vi "TestCloneAPI.vi"() -> ()   [LabVIEW 2018, in "DigitizerModule.lvlib"]
uses:
  DigitizerModule.lvlib
  DigitizerPlugins/DigitizerBaseClass/Typedefs/WfrmAttributes.ctl
  TestInfo.ctl
  <userlib>/NIST/ModuleAdminLib/CloneRegistration/CloneRegistration.lvclass
  <userlib>/NIST/ModuleAdminLib/ModuleAdmin/ModuleAdmin.lvclass/ModuleAdmin.ctl
  <userlib>/NIST/ModuleAdminLib/ModuleAdmin/ModuleAdmin.lvclass
  PublicAPI/Arguments/Broadcasts/clDidInit.ctl
  PublicAPI/Arguments/Requests/clStopArgument.ctl
  <userlib>/NIST/ModuleAdminLib/ModuleAdmin/Accessors/Read CloneRegRef.vi
  <userlib>/NIST/ModuleAdminLib/ModuleAdmin/Accessors/Write CloneRegRef.vi
  DigitizerPlugins/DigitizerBaseClass/DigitizerBase.lvclass
panel:
  in  "btnClose":bool
  out "Attributes":T1[][](array[typedef])
  out "Timing":cluster{"Time Stamp":timestamp, "dt":dbl}[][](array[cluster])
  in  "btnAbort":bool
  in  "btnClear":bool
  in  "btnCfgTrig":bool
  in  "btnCfgAquis":bool
  in  "btnCfgChan":bool
  out "Waveform Chart":waveform(dbl)[](graph)
  in  "btnInitialize":bool
  in  "btnReadWfrm":bool
  in  "btnFetch":bool
  in  "btnPref":bool
  in  "Show Panel":bool=TRUE
  in  "Plugin Type":u16(ring) items=["Agilent3458", "IVI Digitizer", "AbsPhase_Voltage", "Analyse Waveforms", "Debug", "INRiM_3Ch", "INRiM_4Ch", "INRiM_5Ch", "INRiM_6Ch", "INRM_1Ch", "Offset Trigger", "PMU Cal", "PRS_FGen", "Simulation"]
  in  "btnLoadPlugin":bool
  out "Path":path
  in  "btnRequestINIPath":bool
  in  "btnRemove":bool
  out "Status Log":string
  out "Active Modules (Array)":string[](array[string])
  in  "btnAdd":bool
  in  "btnStop":bool
  in  "Select Module":i32(ring)=-1 caption="Select Module to send Request" items=["All"=-1]
  # "Hidden"
  # "Visible"
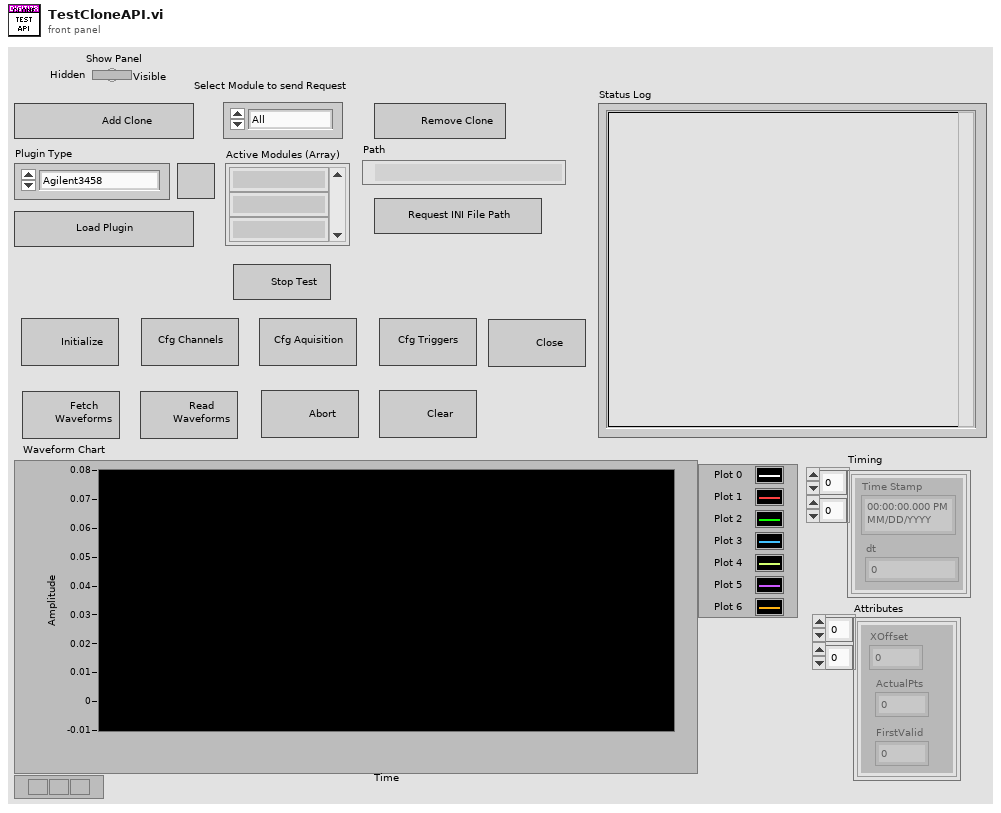
[diagram p1: front panel]
types:
  T1 = typedef "DigitizerPlugins.lvlib/DigitizerBase.lvclass/WfrmAttributes.ctl" = cluster{"XOffset":dbl, "ActualPts":i64, "FirstValid":i64}
  T2 = typedef "DigitizerModule.lvlib/TestInfo.ctl" = cluster{"PluginIniFilePaths":path[]}
  T3 = typedef "DigitizerModule.lvlib/clBroadcastEvents.ctl" = cluster{"DidInit":refnum<user-event>, "StatusUpdate":refnum<user-event>, "ErrorReport":refnum<user-event>, "DidStop":refnum<user-event>, "PathToINI":refnum<user-event>, "Channels":refnum<user-event>, "Acq":refnum<user-event>, "Trigger":refnum<user-event>, "Waveforms":refnum<user-event>}
  T4 = typedef "DigitizerModule.lvlib/clDidInit.ctl" = cluster{"Init?":bool, "ModuleAdmin":refnum<class "ModuleAdmin.lvclass">}
  T5 = typedef "DigitizerModule.lvlib/clStopArgument.ctl" = cluster{"Exit via Stop Module Req?":bool, "Wait for Module to stop?":bool, "ModuleAdmin":refnum<class "ModuleAdmin.lvclass">}
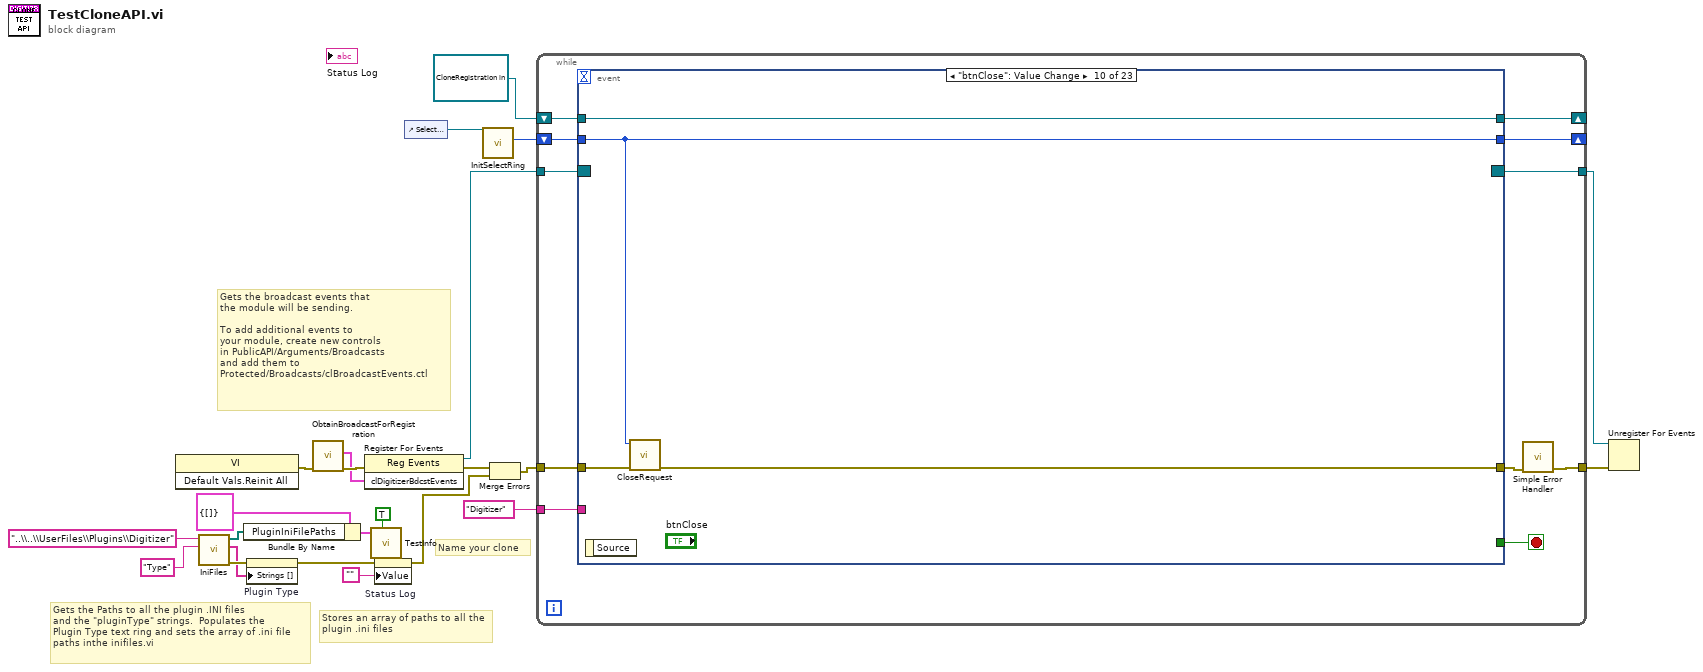
[diagram p0: block diagram]
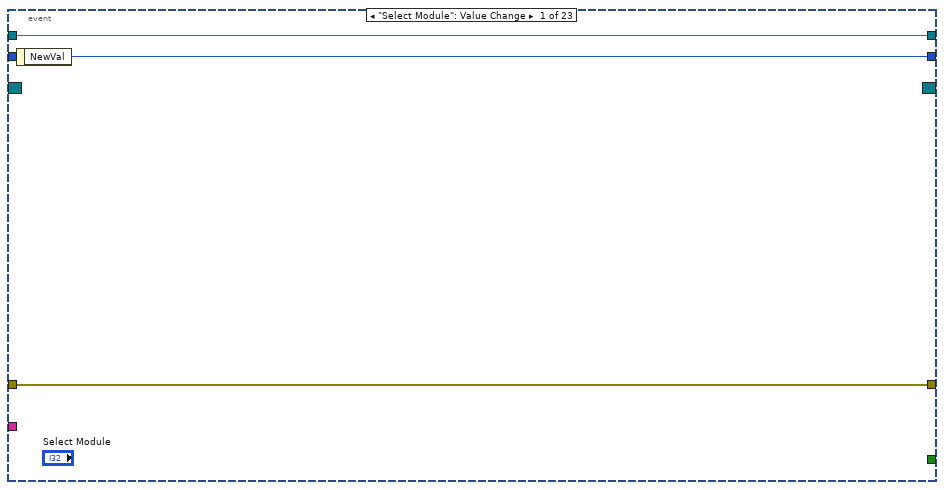
[diagram p2: hidden frame]
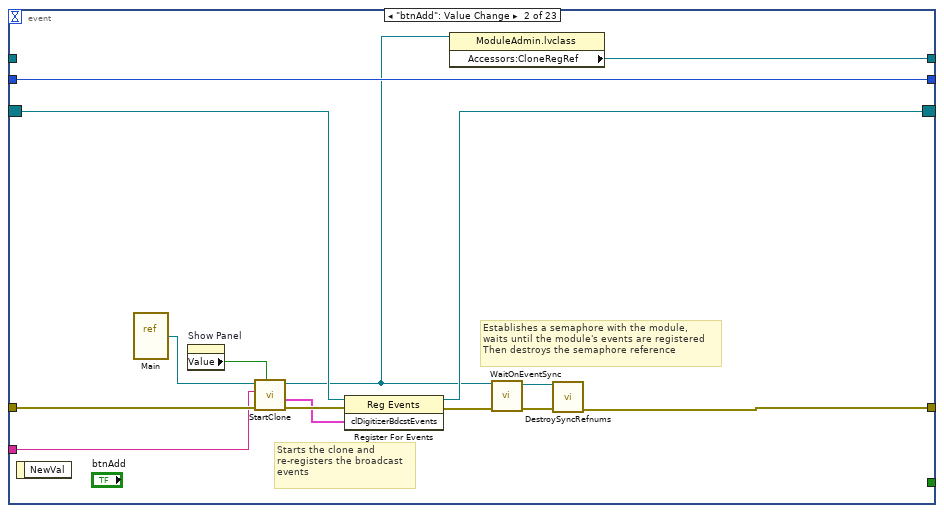
[diagram p3: hidden frame]
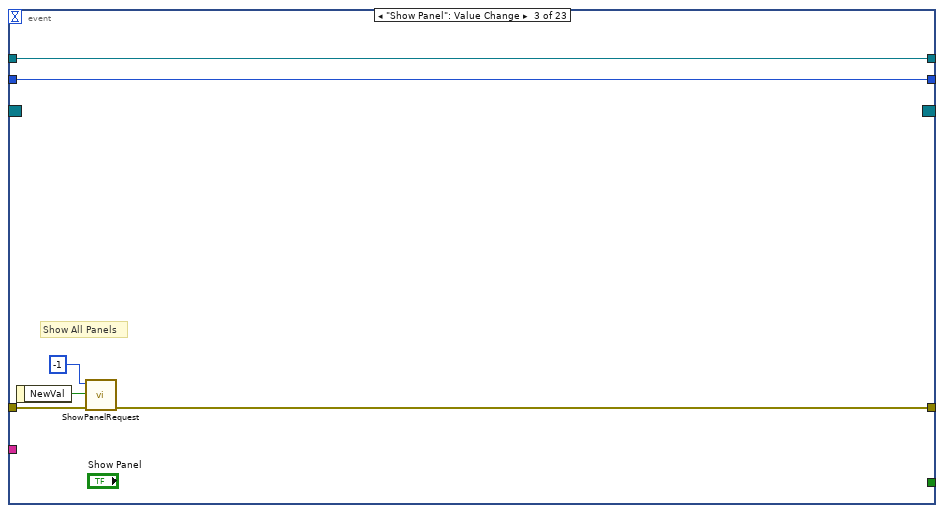
[diagram p4: hidden frame]
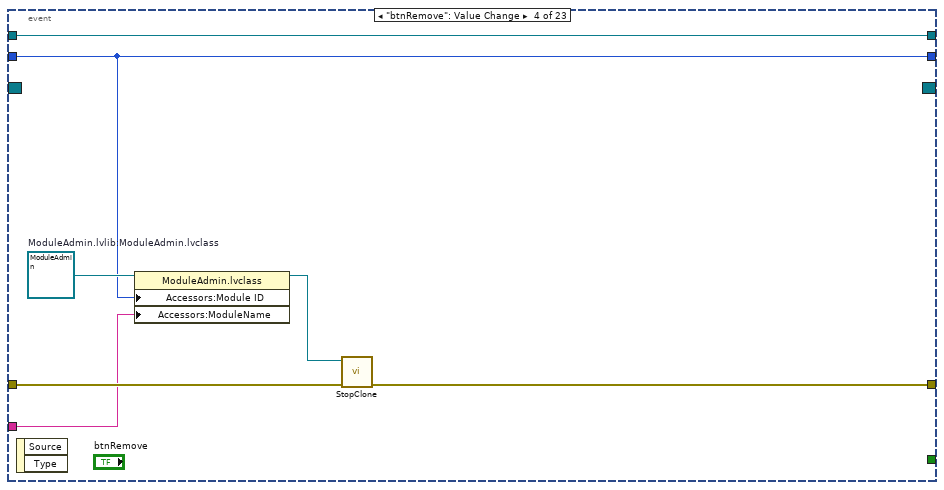
[diagram p5: hidden frame]
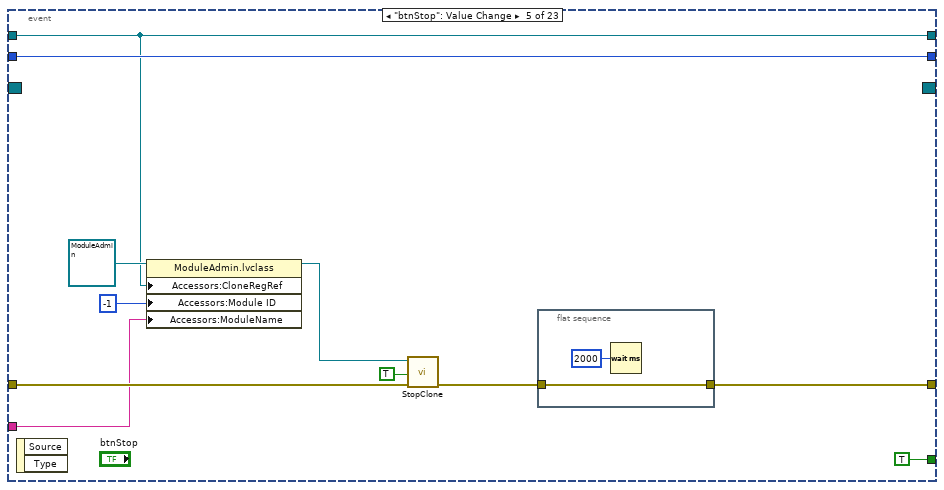
[diagram p6: hidden frame]
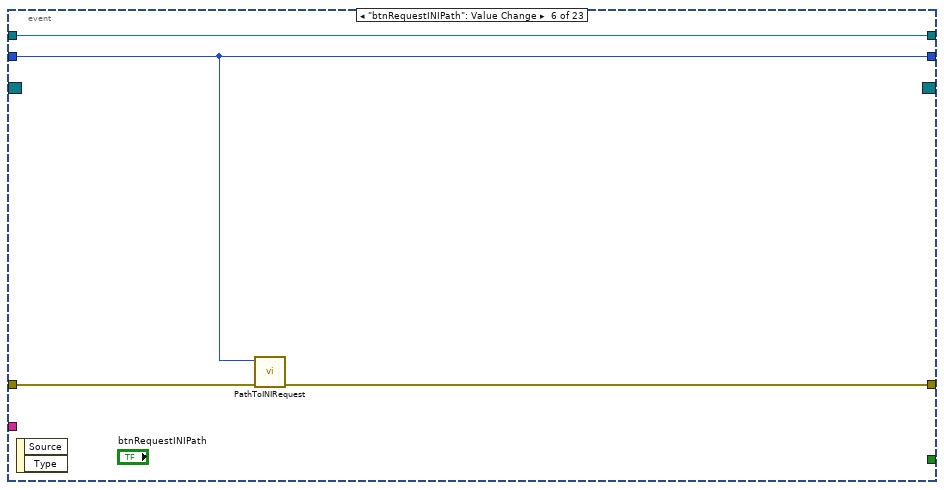
[diagram p7: hidden frame]
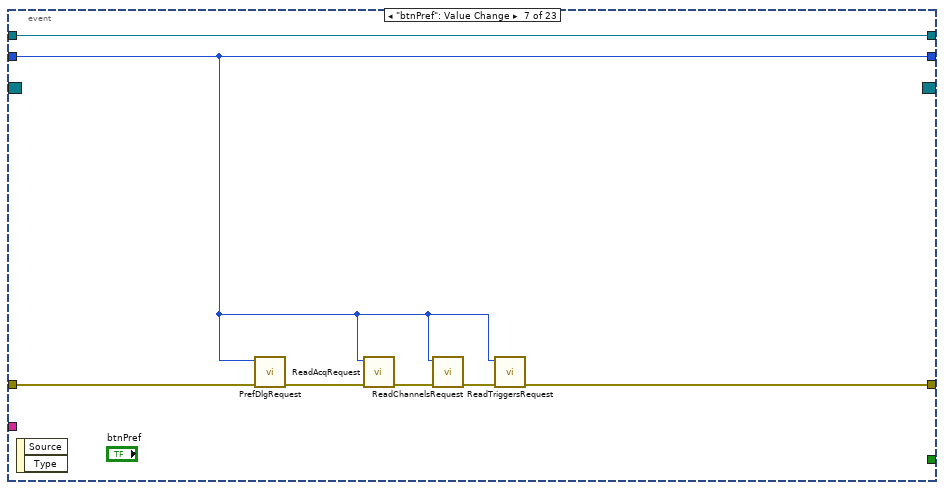
[diagram p8: hidden frame]
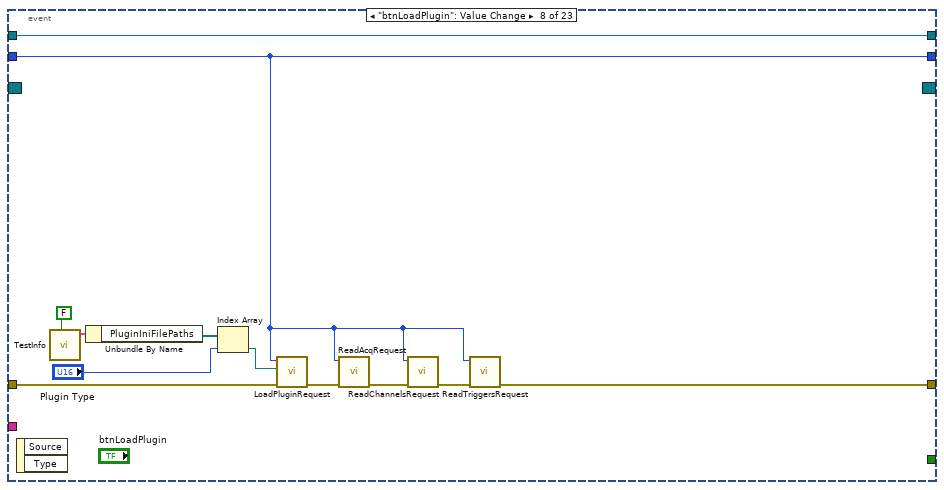
[diagram p9: hidden frame]
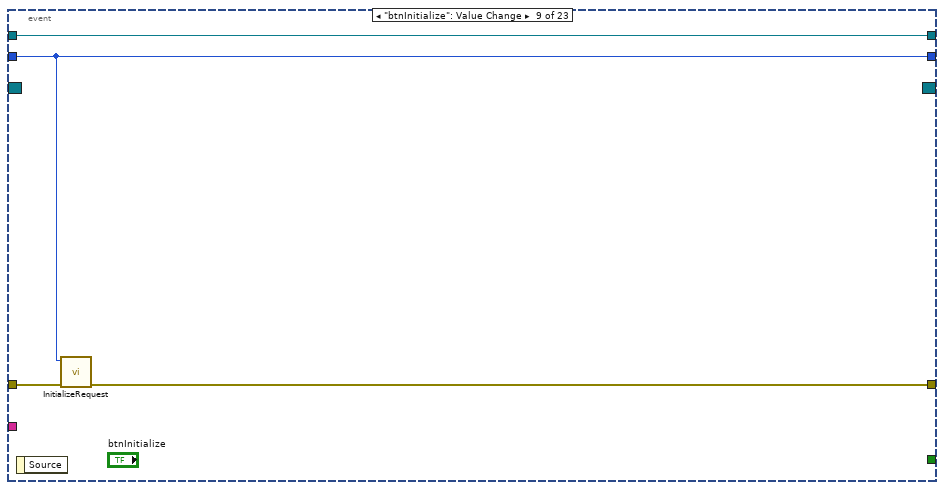
[diagram p10: hidden frame]
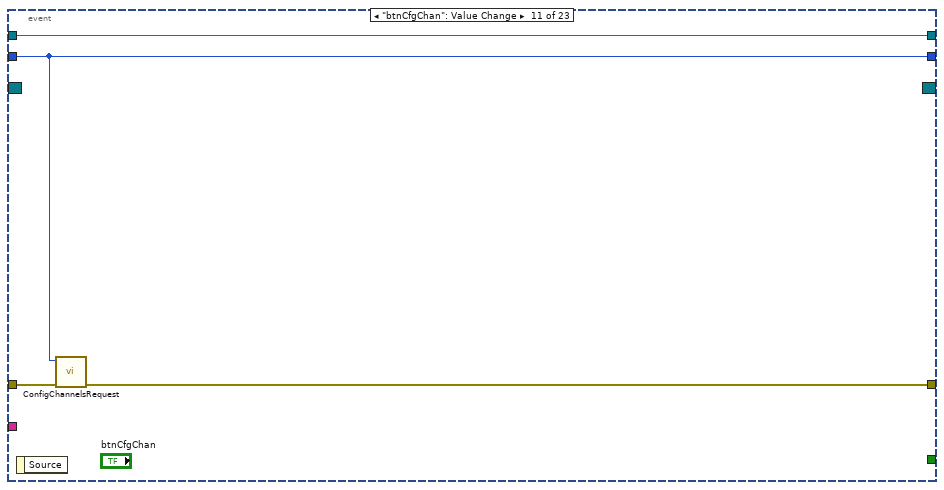
[diagram p11: hidden frame]
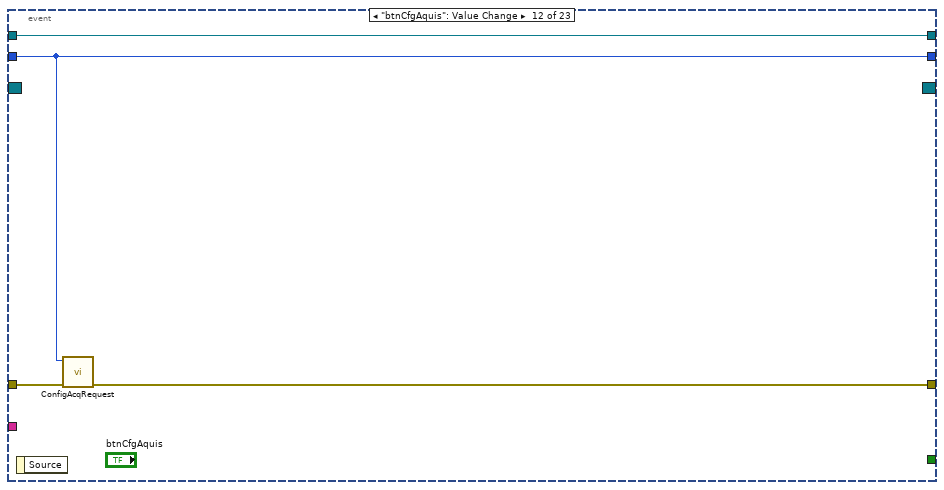
[diagram p12: hidden frame]
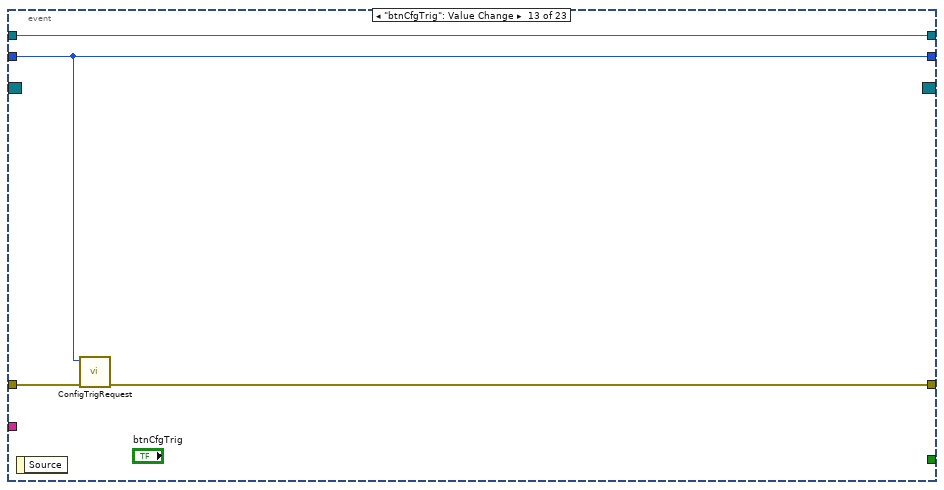
[diagram p13: hidden frame]
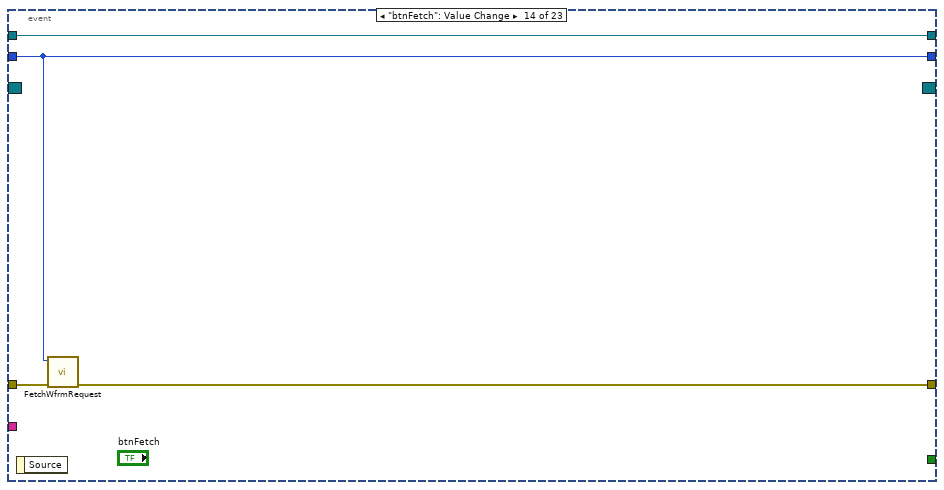
[diagram p14: hidden frame]
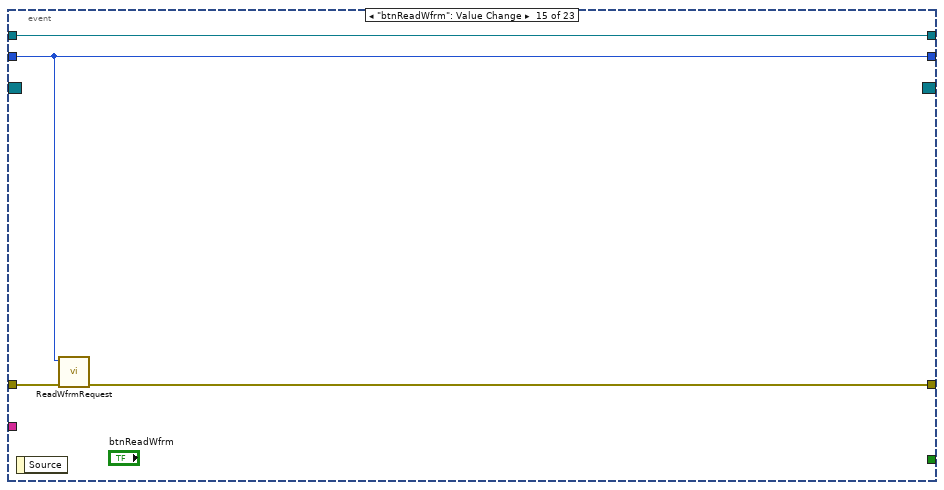
[diagram p15: hidden frame]
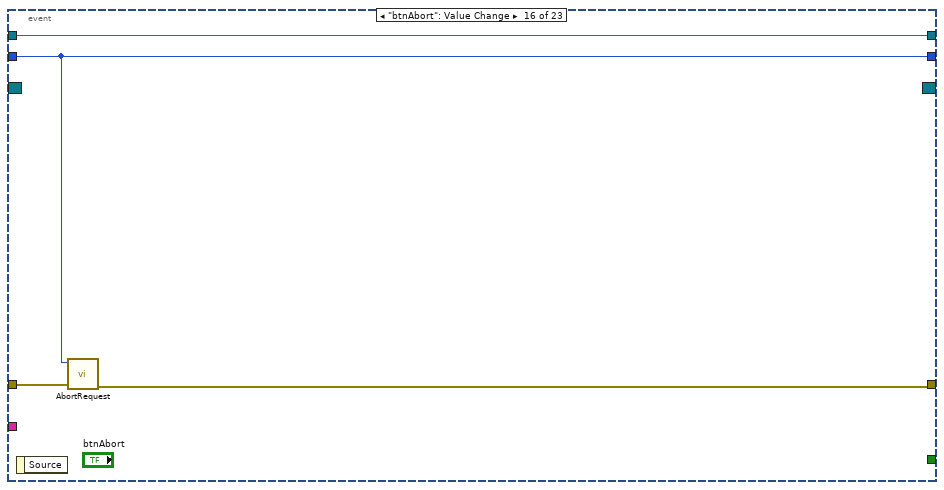
[diagram p16: hidden frame]
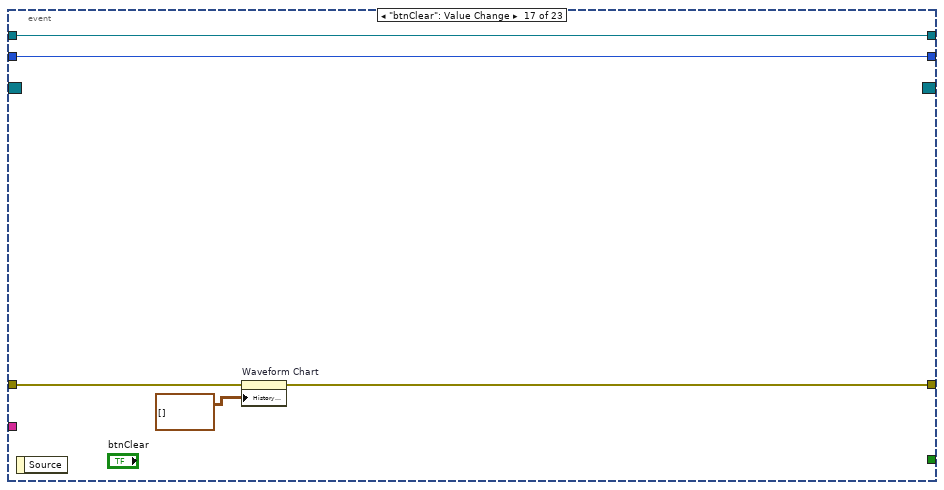
[diagram p17: hidden frame]
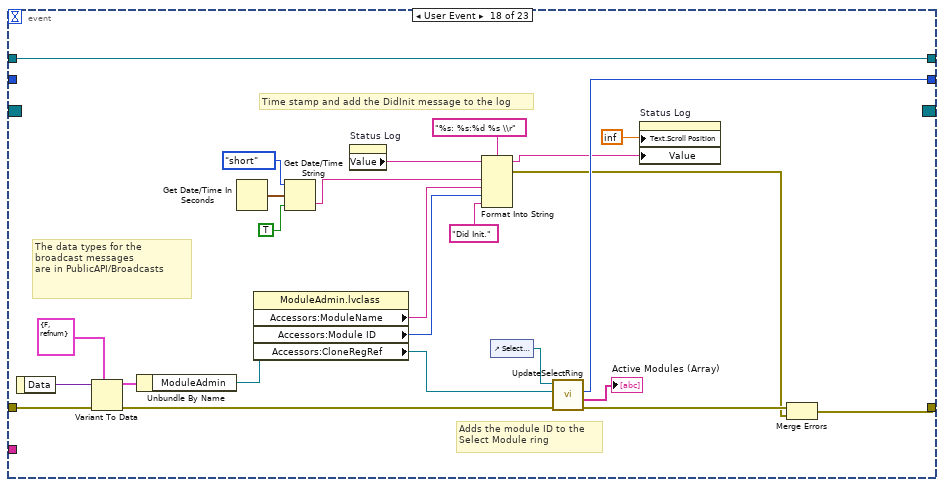
[diagram p18: hidden frame]
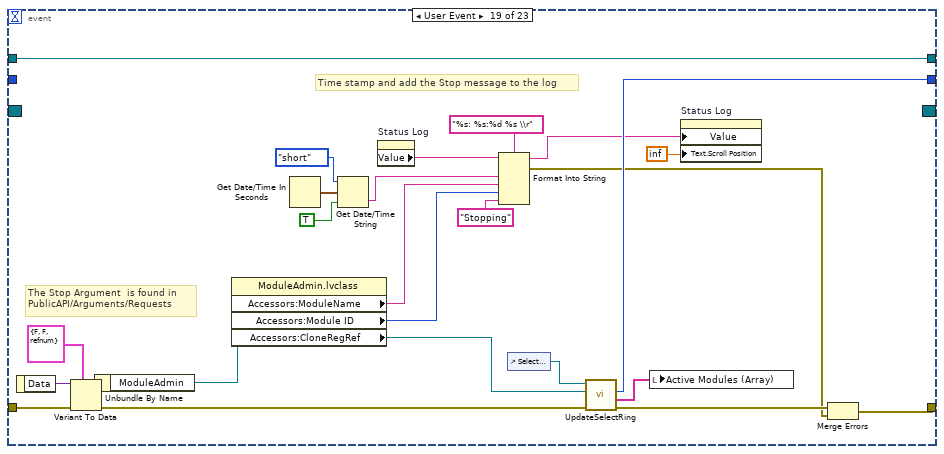
[diagram p19: hidden frame]
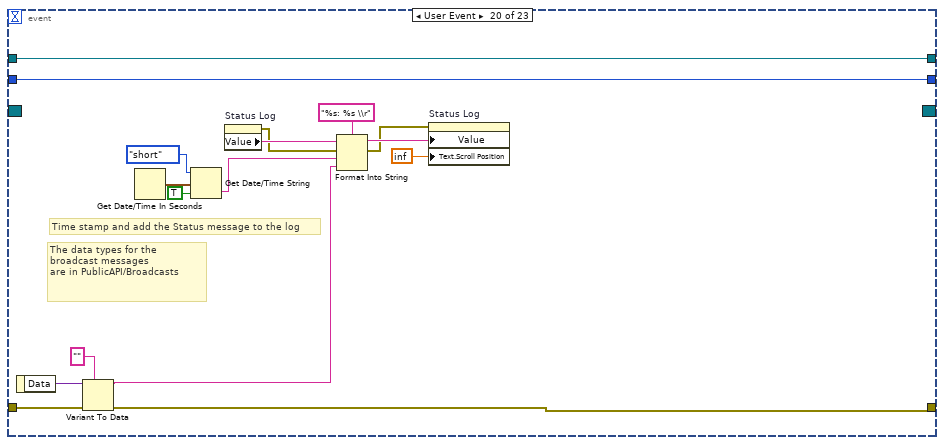
[diagram p20: hidden frame]
diagram:
  # "Stores an array of paths to all the plugin .ini files"
  # "Gets the Paths to all the plugin .INI files\nand the \"pluginType\" strings.  Populates the \nPlugin Type text ring and sets the array of .ini file\npaths inthe inifiles.vi"
  # "Name your clone"
  # "Gets the broadcast events that\nthe module will be sending.\n\nTo add additional events to\nyour module, create new controls\nin PublicAPI/Arguments/Broadcasts\nand add them to\nProtected/Broadcasts/clBroadcastEvents.ctl"
  n1 = invoke class="VI" method="Default Vals.Reinit All"() -> (error out=w21:errorcluster)  [unwired: 3 in, 2 out]
  n2 = call "IniFiles.vi"("iniKey"="Type", "name or relative path"="..\\..\\UserFiles\\Plugins\\Digitizer") -> ("error out"=w15:errorcluster, "Types"=w14:string[], "IniFilePaths"=w13:path[])  [unwired: 7 in]
  n3 = Bundle By Name(cluster=T2 {"PluginIniFilePaths"=[]} ("TestInfo"), "PluginIniFilePaths"=w13) -> (w12:T2)
  n4 = property on="Plugin Type" class="Ring (strict)"(error in=w15, "Strings []"=w14) -> (error out=w3:errorcluster)  [unwired: 1 in, 1 out]
  n5 = call "ObtainBroadcastForRegistration.vi"("error in (no error)"=w21) -> ("error out"=w20:errorcluster, "clDigitizerBdcstEvents"=w19:T3)  [unwired: 9 in]
  n6 = register-events(error in=w20, w19) -> (reference out=w17:refnum<event-registration>, error out=w18:errorcluster)  [unwired: 1 in]
  n7 = call "TestInfo.vi"("Set (f)"=TRUE, "TestInfo 2"=w12) -> ()  [unwired: 9 in, 1 out]
  n8 = property on="Status Log" class="Str"(error in=w3, "Value"="") -> (error out=w2:errorcluster)  [unwired: 1 in, 1 out]
  n9 = control-ref of="Select Module"() -> (w23:refnum<vi>)
  n10 = call "InitSelectRing.vi"("Ring Refnum"=w23) -> ("Module Ring Value"=w22:i32)  [unwired: 9 in, 1 out]
  n11 = Merge Errors(w18, w2) -> (w10:errorcluster)
  n12 = while {
    shift-right: [w33] -> _
    shift-left: w22 -> [w34]
    tunnel: w10 -> [w31]
    tunnel: w17 -> [w28]
    tunnel: [w29] -> w6
    tunnel: "Digitizer" ("ModuleName") -> [w27]
    tunnel: [w26] -> w5
    shift-right: [w25] -> _
    shift-left: refnum<data-value> refnum ("Accessors:CloneRegRef") -> [w24]
    stop <- w32 stop-if-true
    n13 = event shown="[9] \"btnClose\": Value Change" {
      selector: w28 -> [_ w44 _ _ _ _ _ _ _ _ _ _ _ _ _ _ _ _ _ _ _ _ _]
      dyn-events: [_ w43 _ _ _ _ _ _ _ _ _ _ _ _ _ _ _ _ _ _ _ _ _] -> w26
      timeout: _ -> [_ _ _ _ _ _ _ _ _ _ _ _ _ _ _ _ _ _ _ _ _ _ _]
      tunnel: w34 -> [_ w52 w54 w62 w76 w82 w83 w90 w102 w106 w112 w116 w118 w122 w126 w132 w137 _ _ w205 w208 w221 w231]
      tunnel: [w37 w52 w54 w62 w76 w82 w83 w90 w102 w106 w112 w116 w118 w122 w126 w132 w137 w158 w177 w205 w208 w221 w231] -> w33
      tunnel: [_ _ _ _ TRUE _ _ _ _ _ _ _ _ _ _ _ _ _ _ _ _ _ _] -> w32
      tunnel: w31 -> [w36 w51 w57 w65 w74 w81 w89 w101 w105 w109 w113 w117 w120 w125 w129 w133 w136 w163 w184 w203 w213 w217 w234]
      tunnel: [w36 w45 w55 w64 w66 w80 w84 w91 w104 w108 w110 w114 w119 w124 w128 w130 w135 w149 w174 w189 w212 w216 w222] -> w30
      tunnel: w27 -> [_ w41 _ w61 w71 _ _ _ _ _ _ _ _ _ _ _ _ _ _ _ _ _ _]
      tunnel: [w35 w38 w53 w59 w68 w79 w88 w95 w103 w107 w111 w115 w121 w123 w127 w131 w138 w142 w167 w195 w206 w215 w232] -> w25
      tunnel: w24 -> [w35 _ w53 w59 w68 w79 w88 w95 w103 w107 w111 w115 w121 w123 w127 w131 w138 w142 w167 w195 w206 w215 w232]
      event "Select Module": Value Change {
        n14 = event-data() -> ("NewVal"=w37:i32)  [unwired: 1 in]
      }
      event "btnAdd": Value Change {
        # "Establishes a semaphore with the module,\nwaits until the module's events are registered\nThen destroys the semaphore reference"
        # "Starts the clone and\nre-registers the broadcast \nevents"
        n15 = event-data() -> ()  [unwired: 1 in, 1 out]
        n16 = vi-ref "Main.vi"() -> (w42:refnum<vi>)
        n17 = property on="Show Panel" class="Bool (strict)"() -> ("Value"=w40:bool)  [unwired: 2 in, 2 out]
        n18 = call "StartClone.vi"("ShowPanel? (f)"=w40, "error in (no error)"=w51, "ModuleName"=w41, "VI Refnum"=w42) -> ("error out"=w50:errorcluster, "clBroadcastEvents"=w46:T3, "ModuleAdmin"=w39:refnum<class "ModuleAdmin.lvclass">)  [unwired: 5 in]
        n19 = register-events(reference=w44, error in=w50, w46) -> (reference out=w43:refnum<event-registration>, error out=w49:errorcluster)
        n20 = property class="ModuleAdmin.lvclass"(reference=w39) -> ("Accessors:CloneRegRef"=w38:refnum<data-value>)  [unwired: 1 in, 2 out]
        n21 = call <userlib>:"WaitOnEventSync.vi"("error in (no error)"=w49, "ModuleAdmin"=w39) -> ("error out"=w48:errorcluster, "ModuleAdmin"=w47:refnum<class "ModuleAdmin.lvclass">)  [unwired: 8 in]
        n22 = call <userlib>:"DestroySyncRefnums.vi"("error in (no error)"=w48, "ModuleAdmin"=w47) -> ("error out"=w45:errorcluster)  [unwired: 9 in]
      }
      event "Show Panel": Value Change {
        # "Show All Panels"
        n23 = event-data() -> ("NewVal"=w58:bool)  [unwired: 1 in]
        n24 = call "ShowPanelRequest.vi"("error in (no error)"=w57, "ShowPanel?"=w58, "ModuleID"=-1) -> ("error out"=w55:errorcluster)  [unwired: 8 in]
      }
      event "btnRemove": Value Change {
        w63 = refnum<class "ModuleAdmin.lvclass"> refnum  # ModuleAdmin.lvlib:ModuleAdmin.lvclass
        n25 = event-data() -> ()  [unwired: 1 in, 2 out]
        n26 = property class="ModuleAdmin.lvclass"(reference=w63, "Accessors:Module ID"=w62, "Accessors:ModuleName"=w61) -> (reference out=w60:refnum<class "ModuleAdmin.lvclass">)  [unwired: 1 in, 1 out]
        n27 = call "StopClone.vi"("error in (no error)"=w65, "ModuleAdmin"=w60) -> ("error out"=w64:errorcluster)  [unwired: 9 in]
      }
      event "btnStop": Value Change {
        n28 = event-data() -> ()  [unwired: 1 in, 2 out]
        n29 = property class="ModuleAdmin.lvclass"(reference=refnum<class "ModuleAdmin.lvclass"> refnum ("ModuleAdmin.lvlib:ModuleAdmin.lvclass"), "Accessors:CloneRegRef"=w68, "Accessors:Module ID"=-1 ("Module ID"), "Accessors:ModuleName"=w71) -> (reference out=w70:refnum<class "ModuleAdmin.lvclass">)  [unwired: 1 in, 1 out]
        n30 = call "StopClone.vi"("error in (no error)"=w74, "Wait for Module to stop?"=TRUE, "ModuleAdmin"=w70) -> ("error out"=w67:errorcluster)  [unwired: 8 in]
        n31 = flat-sequence {
          tunnel: w67 -> [w77]
          tunnel: [w77] -> w66
          frame #0 {
            n32 = Wait (ms)(milliseconds to wait=u32 2000) -> ()  [unwired: 1 out]
          }
        }
      }
      event "btnRequestINIPath": Value Change {
        n33 = event-data() -> ()  [unwired: 1 in, 2 out]
        n34 = call "PathToINIRequest.vi"("error in (no error)"=w81, "ModuleID"=w82) -> ("error out"=w80:errorcluster)  [unwired: 9 in]
      }
      event "btnPref": Value Change {
        n35 = event-data() -> ()  [unwired: 1 in, 2 out]
        n36 = call "PrefDlgRequest.vi"("error in (no error)"=w89, "ModuleID"=w83) -> ("error out"=w87:errorcluster)  [unwired: 9 in]
        n37 = call "ReadAcqRequest.vi"("error in (no error)"=w87, "ModuleID"=w83) -> ("error out"=w86:errorcluster)  [unwired: 9 in]
        n38 = call "ReadChannelsRequest.vi"("error in (no error)"=w86, "ModuleID"=w83) -> ("error out"=w85:errorcluster)  [unwired: 9 in]
        n39 = call "ReadTriggersRequest.vi"("error in (no error)"=w85, "ModuleID"=w83) -> ("error out"=w84:errorcluster)  [unwired: 9 in]
      }
      event "btnLoadPlugin": Value Change {
        n40 = event-data() -> ()  [unwired: 1 in, 2 out]
        n41 = call "TestInfo.vi"("Set (f)"=FALSE) -> ("TestInfo"=w99:T2)  [unwired: 10 in]
        n42 = Unbundle By Name(w99) -> ("PluginIniFilePaths"=w98:path[])
        n43 = Index Array(array=w98, index="Plugin Type") -> (element=w96:path)
        n44 = call "LoadPluginRequest.vi"("error in (no error)"=w101, "PathToPluginINI"=w96, "ModuleID"=w90) -> ("error out"=w94:errorcluster)  [unwired: 8 in]
        n45 = call "ReadAcqRequest.vi"("error in (no error)"=w94, "ModuleID"=w90) -> ("error out"=w93:errorcluster)  [unwired: 9 in]
        n46 = call "ReadChannelsRequest.vi"("error in (no error)"=w93, "ModuleID"=w90) -> ("error out"=w92:errorcluster)  [unwired: 9 in]
        n47 = call "ReadTriggersRequest.vi"("error in (no error)"=w92, "ModuleID"=w90) -> ("error out"=w91:errorcluster)  [unwired: 9 in]
      }
      event "btnInitialize": Value Change {
        n48 = event-data() -> ()  [unwired: 1 in, 1 out]
        n49 = call "InitializeRequest.vi"("error in (no error)"=w105, "ModuleID"=w102) -> ("error out"=w104:errorcluster)  [unwired: 9 in]
      }
      event "btnClose": Value Change {
        n50 = event-data() -> ()  [unwired: 1 in, 1 out]
        n51 = call "CloseRequest.vi"("error in (no error)"=w109, "ModuleID"=w106) -> ("error out"=w108:errorcluster)  [unwired: 9 in]
      }
      event "btnCfgChan": Value Change {
        n52 = event-data() -> ()  [unwired: 1 in, 1 out]
        n53 = call "ConfigChannelsRequest.vi"("error in (no error)"=w113, "ModuleID"=w112) -> ("error out"=w110:errorcluster)  [unwired: 9 in]
      }
      event "btnCfgAquis": Value Change {
        n54 = event-data() -> ()  [unwired: 1 in, 1 out]
        n55 = call "ConfigAcqRequest.vi"("error in (no error)"=w117, "ModuleID"=w116) -> ("error out"=w114:errorcluster)  [unwired: 9 in]
      }
      event "btnCfgTrig": Value Change {
        n56 = event-data() -> ()  [unwired: 1 in, 1 out]
        n57 = call "ConfigTrigRequest.vi"("error in (no error)"=w120, "ModuleID"=w118) -> ("error out"=w119:errorcluster)  [unwired: 9 in]
      }
      event "btnFetch": Value Change {
        n58 = event-data() -> ()  [unwired: 1 in, 1 out]
        n59 = call "FetchWfrmRequest.vi"("error in (no error)"=w125, "ModuleID"=w122) -> ("error out"=w124:errorcluster)  [unwired: 9 in]
      }
      event "btnReadWfrm": Value Change {
        n60 = event-data() -> ()  [unwired: 1 in, 1 out]
        n61 = call "ReadWfrmRequest.vi"("error in (no error)"=w129, "ModuleID"=w126) -> ("error out"=w128:errorcluster)  [unwired: 9 in]
      }
      event "btnAbort": Value Change {
        n62 = event-data() -> ()  [unwired: 1 in, 1 out]
        n63 = call "AbortRequest.vi"("error in (no error)"=w133, "ModuleID"=w132) -> ("error out"=w130:errorcluster)  [unwired: 9 in]
      }
      event "btnClear": Value Change {
        n64 = event-data() -> ()  [unwired: 1 in, 1 out]
        n65 = property on="Waveform Chart" class="WFChart (strict)"(error in=w136, "History Data"=waveform(dbl)[][] []) -> (error out=w135:errorcluster)  [unwired: 1 in, 1 out]
      }
      event User Event {
        # "Adds the module ID to the \nSelect Module ring"
        # "Time stamp and add the DidInit message to the log"
        # "The data types for the broadcast messages\nare in PublicAPI/Broadcasts"
        n66 = event-data() -> ("Data"=w162:variant)  [unwired: 1 in]
        n67 = Variant To Data(error in=w163, type=T4 {"Init?"=FALSE, "ModuleAdmin"=refnum} ("clDidInit"), Variant=w162) -> (data=w155:T4, error out=w160:errorcluster)
        n68 = Unbundle By Name(w155) -> ("ModuleAdmin"=w147:refnum<class "ModuleAdmin.lvclass">)
        n69 = Get Date/Time In Seconds() -> (seconds since 1Jan1904=w153:timestamp)
        n70 = property class="ModuleAdmin.lvclass"(reference=w147) -> ("Accessors:ModuleName"=w145:string, "Accessors:Module ID"=w144:i32, "Accessors:CloneRegRef"=w143:refnum<data-value>)  [unwired: 1 in, 2 out]
        n71 = Get Date/Time String(date format (0)=enum16{"short", "long", "abbreviated"}."short", seconds (now)=w153, want seconds? (F)=TRUE) -> (time string=w156:string)  [unwired: 1 out]
        n72 = property on="Status Log" class="Str"() -> ("Value"=w141:string)  [unwired: 2 in, 2 out]
        n73 = Format Into String(format string="%s: %s:%d %s \\r", initial string=w141, w156, w145, w144, "Did Init.") -> (resulting string=w140:string, error out=w150:errorcluster)  [unwired: 1 in]
        n74 = control-ref of="Select Module"() -> (w159:refnum<vi>)
        n75 = call "UpdateSelectRing.vi"("error in (no error)"=w160, "CloneRegRef"=w143, "Ring Refnum"=w159) -> ("error out"=w151:errorcluster, "ActiveModules"=→"Active Modules (Array)":string[], "Module Ring Value"=w158:i32)  [unwired: 6 in]
        n76 = property on="Status Log" class="Str"("Text.Scroll Position"=inf, "Value"=w140) -> ()  [unwired: 2 in, 2 out]
        n77 = Merge Errors(w151, w150) -> (w149:errorcluster)
      }
      event User Event {
        # "Time stamp and add the Stop message to the log"
        # "The Stop Argument  is found in\nPublicAPI/Arguments/Requests"
        n78 = event-data() -> ("Data"=w183:variant)  [unwired: 1 in]
        n79 = Variant To Data(error in=w184, type=T5 {"Exit via Stop Module Req?"=FALSE, "Wait for Module to stop?"=FALSE, "ModuleAdmin"=refnum} ("Stop Argument"), Variant=w183) -> (data=w181:T5, error out=w180:errorcluster)
        n80 = Unbundle By Name(w181) -> ("ModuleAdmin"=w172:refnum<class "ModuleAdmin.lvclass">)
        n81 = property class="ModuleAdmin.lvclass"(reference=w172) -> ("Accessors:ModuleName"=w170:string, "Accessors:Module ID"=w169:i32, "Accessors:CloneRegRef"=w168:refnum<data-value>)  [unwired: 1 in, 2 out]
        n82 = Get Date/Time In Seconds() -> (seconds since 1Jan1904=w186:timestamp)
        n83 = Get Date/Time String(date format (0)=enum16{"short", "long", "abbreviated"}."short", seconds (now)=w186, want seconds? (F)=TRUE) -> (time string=w188:string)  [unwired: 1 out]
        n84 = property on="Status Log" class="Str"() -> ("Value"=w166:string)  [unwired: 2 in, 2 out]
        n85 = Format Into String(format string="%s: %s:%d %s \\r", initial string=w166, w188, w170, w169, "Stopping") -> (resulting string=w165:string, error out=w175:errorcluster)  [unwired: 1 in]
        n86 = control-ref of="Select Module"() -> (w179:refnum<vi>)
        n87 = call "UpdateSelectRing.vi"("error in (no error)"=w180, "CloneRegRef"=w168, "Ring Refnum"=w179) -> ("error out"=w176:errorcluster, "ActiveModules"=w178:string[], "Module Ring Value"=w177:i32)  [unwired: 6 in]
        n88 = local write "Active Modules (Array)"(w178) -> ()
        n89 = property on="Status Log" class="Str"("Value"=w165, "Text.Scroll Position"=inf) -> ()  [unwired: 2 in, 2 out]
        n90 = Merge Errors(w176, w175) -> (w174:errorcluster)
      }
      event User Event {
        # "Time stamp and add the Status message to the log"
        # "The data types for the broadcast messages\nare in PublicAPI/Broadcasts"
        n91 = event-data() -> ("Data"=w202:variant)  [unwired: 1 in]
        n92 = Variant To Data(error in=w203, type="" ("clStatUpdate"), Variant=w202) -> (data=w196:string, error out=w189:errorcluster)
        n93 = Get Date/Time In Seconds() -> (seconds since 1Jan1904=w200:timestamp)
        n94 = Get Date/Time String(date format (0)=enum16{"short", "long", "abbreviated"}."short", seconds (now)=w200, want seconds? (F)=TRUE) -> (time string=w197:string)  [unwired: 1 out]
        n95 = property on="Status Log" class="Str"() -> (error out=w192:errorcluster, "Value"=w194:string)  [unwired: 2 in, 1 out]
        n96 = Format Into String(format string="%s: %s \\r", initial string=w194, error in=w192, w197, w196) -> (resulting string=w193:string, error out=w191:errorcluster)
        n97 = property on="Status Log" class="Str"(error in=w191, "Value"=w193, "Text.Scroll Position"=inf) -> ()  [unwired: 1 in, 2 out]
      }
      event User Event {
        # "#CodeNeeded\nThis is a very crude error handler\nA better error handler will be needed"
        # "The data types for the broadcast messages\nare in PublicAPI/Broadcasts"
        n98 = event-data() -> ("ModuleID"=w210:i32, "Data"=w214:variant)  [unwired: 1 in]
        n99 = Variant To Data(error in=w213, type=errorcluster {"status"=FALSE, "code"=0, "source"=""} ("Cluster"), Variant=w214) -> (data=w207:errorcluster, error out=w212:errorcluster)
        n100 = Number To Decimal String(number=w210) -> (decimal integer string=w209:string)  [unwired: 1 in]
        n101 = call <vilib>:"General Error Handler.vi"("[error source] (\" \")"=w209, "error in (no error)"=w207) -> ()  [unwired: 9 in, 5 out]
      }
      event User Event {
        n102 = event-data() -> ("Data"=w219:variant)  [unwired: 1 in, 1 out]
        n103 = Variant To Data(error in=w217, type=path "" ("Path"), Variant=w219) -> (data=→"Path":path, error out=w216:errorcluster)
      }
      event User Event {
        n104 = event-data() -> ("Data"=w235:variant)  [unwired: 1 in]
        n105 = Variant To Data(error in=w234, type=waveform(dbl)[][] [], Variant=w235) -> (data=w224:waveform(dbl)[][], error out=w223:errorcluster)
        n106 = for {
          tunnel: w224 -> [w240] mode=indexing
          tunnel: [w239] -> w226 mode=indexing
          tunnel: [w238] -> w229 mode=indexing
          shift-right: [w236] -> w222
          shift-left: w223 -> [w237]
          stop <- w236 stop-if-true
          n107 = for {
            tunnel: w240 -> [w250] mode=indexing
            tunnel: [w244] -> w238 mode=indexing
            tunnel: [w243] -> w239 mode=indexing
            tunnel: w237 -> [w242]
            tunnel: [w241] -> w236
            stop <- w241 stop-if-true
            n108 = Unbundle By Name(w250) -> ("t0"=w248:timestamp, "dt"=w247:dbl, "attributes"=w246:variant)
            n109 = Bundle By Name(cluster=cluster{"Time Stamp":timestamp, "dt":dbl} {"Time Stamp"=timestamp(0 s since 1904-01-01), "dt"=0.0} ("Cluster"), "Time Stamp"=w248, "dt"=w247) -> (w244:cluster{"Time Stamp":timestamp, "dt":dbl})
            n110 = Variant To Data(error in=w242, type=T1 {"XOffset"=0.0, "ActualPts"=0, "FirstValid"=0} ("Attributes"), Variant=w246) -> (data=w243:T1, error out=w241:errorcluster)
          }
          "Waveform Chart" <- w240
        }
        n111 = property on="Timing" class="Arr (strict)"() -> ("Value"=w230:cluster{"Time Stamp":timestamp, "dt":dbl}[][])  [unwired: 2 in, 2 out]
        n112 = property on="Attributes" class="Arr (strict)"() -> ("Value"=w227:T1[][])  [unwired: 2 in, 2 out]
        n113 = Build Array (concatenate)(w230, w229) -> (→"Timing":cluster{"Time Stamp":timestamp, "dt":dbl}[][])
        n114 = Build Array (concatenate)(w227, w226) -> (→"Attributes":T1[][])
      }
    }
    n115 = call <vilib>:"Simple Error Handler.vi"("error in (no error)"=w30) -> ("error out"=w29:errorcluster)  [unwired: 4 in, 4 out]
  }
  n116 = Unregister For Events(event registration refnum=w5, error in=w6) -> ()  [unwired: 1 out]
